vi "RSZVB Set Port Waveguide Attenuator Offset.vi"(7 "Offset (0)":i32, 8 "error in (no error)":errorcluster {"code" format="%.0x"}, 9 "Port (1)":i32=1, 10 "Channel (1)":i32=1, 11 "VISA session":refnum<visa-resource-name>) -> (0 "error out":errorcluster {"code" format="%.0x"}, 3 "dup VISA session":refnum<visa-resource-name>)   [LabVIEW 2011]
doc: "This VI specifies the offset factor for the linear power transfer model with 0 dB waveguide attenuation.\n\nRemote-control command(s):\nSOURce<Ch>:POWer<Pt>:CONVerter:TRANsfer:OFFSet <offset>"
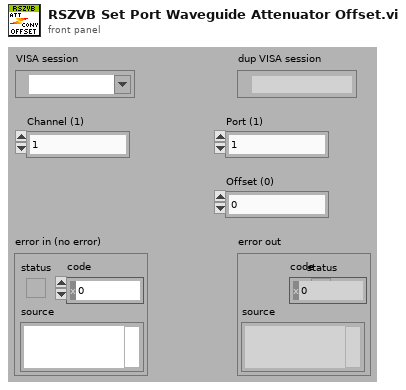
[diagram p1: front panel]
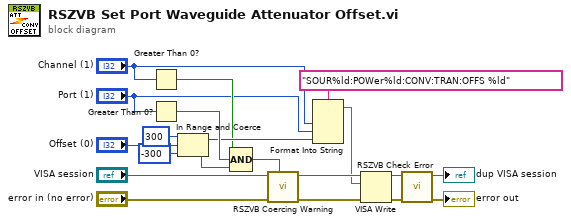
[diagram p0: block diagram]
diagram:
  n1 = Greater Than 0?(x="Channel (1)") -> (x > 0?=w8:bool)
  n2 = Greater Than 0?(x="Port (1)") -> (x > 0?=w14:bool)
  n3 = In Range and Coerce(upper limit=300, x="Offset (0)", lower limit=-300) -> (coerced(x)=w9:i32, In Range?=w15:bool)
  n4 = Compound Arithmetic op=AND(w8, w14, w15) -> (w13:bool)
  n5 = call "RSZVB Coercing Warning.vi"("In Range?"=w13, "error in (no error)"="error in (no error)", "VISA session"="VISA session") -> ("error out"=w18:errorcluster, "dup VISA session"=w19:refnum<visa-resource-name>)  [unwired: 7 in]
  n6 = Format Into String(format string="SOUR%ld:POWer%ld:CONV:TRAN:OFFS %ld", "Channel (1)", "Port (1)", w9) -> (resulting string=w12:string)  [unwired: 2 in, 1 out]
  n7 = VISA Write(VISA resource name=w19, write buffer=w12, error in (no error)=w18) -> (VISA resource name out=w16:refnum<visa-resource-name>, error out=w17:errorcluster)  [unwired: 1 out]
  n8 = call "RSZVB Check Error.vi"("error in (no error)"=w17, "VISA session"=w16) -> ("error out"=→"error out":errorcluster, "dup VISA session"=→"dup VISA session":refnum<visa-resource-name>)  [unwired: 8 in]
